vi "Start Continuous Output.vi"(0 "VISA resource name":refnum<visa-resource-name>, 7 "Continuous Measurement Type (Raw Accelerometer and Angular Rate)":u16(ring) items=["Raw Accelerometer and Angular Rate", "DeltaAngle & DeltaVelocity", "Orientation Matrix", "Orientation Update Matrix", "Acceleration, Angular Rate & Magnetometer Vectors", "Euler Angles", "Temperatures", "Gyro Stabilized Acceleration, Angular Rate & Magnetometer"], 11 "error in (no error)":errorcluster) -> (4 "VISA resource name out":refnum<visa-resource-name>, 15 "error out":errorcluster)   [LabVIEW 2012, in "MicroStrain 3DM-GXx.lvlib"]
doc: "Start continuous output of the specified measurement type."
uses:
  <instrlib>/MicroStrain 3DM-GXx/MicroStrain 3DM-GXx.lvlib
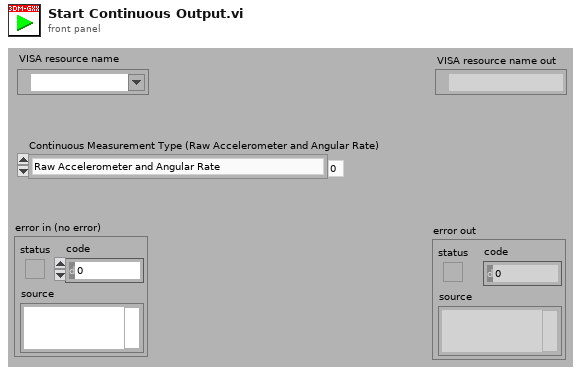
[diagram p1: front panel]
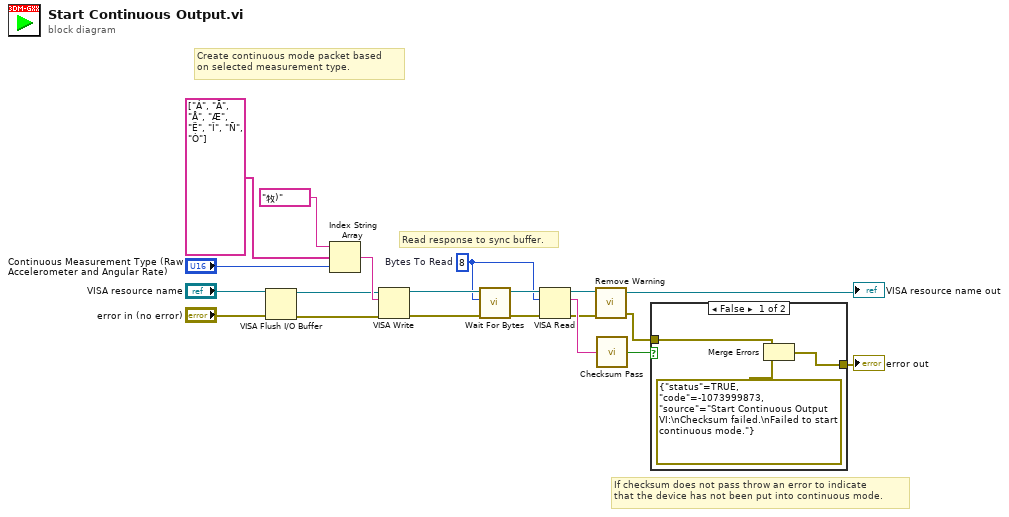
[diagram p0: block diagram]
diagram:
  w16 = u32 8  # Bytes To Read
  # "If checksum does not pass throw an error to indicate \nthat the device has not been put into continuous mode."
  # "Read response to sync buffer."
  # "Create continuous mode packet based \non selected measurement type."
  n1 = VISA Flush I/O Buffer(VISA resource name="VISA resource name", error in (no error)="error in (no error)") -> (VISA resource name out=w2:refnum<visa-resource-name>, error out=w1:errorcluster)  [unwired: 1 in]
  n2 = Index String Array(1:"Continuous Measurement Type (Raw Accelerometer and Angular Rate)", 2:string[] ["Á", "Ã", "Å", "Æ", "Ë", "Î", "Ñ", "Ò"] ("string array"), 3:"牧)" ("write buffer")) -> (0:w5:string)
  n3 = VISA Write(VISA resource name=w2, write buffer=w5, error in (no error)=w1) -> (VISA resource name out=w20:refnum<visa-resource-name>, error out=w19:errorcluster)  [unwired: 1 out]
  n4 = call <instrlib>:"Wait For Bytes.vi"("error in (no error)"=w19, "Bytes To Read (0)"=w16, "VISA resource name"=w20) -> ("error out"=w18:errorcluster, "VISA resource name out"=w17:refnum<visa-resource-name>)  [unwired: 7 in]
  n5 = VISA Read(VISA resource name=w17, byte count=w16, error in (no error)=w18) -> (VISA resource name out=w10:refnum<visa-resource-name>, read buffer=w15:string, error out=w11:errorcluster)  [unwired: 1 out]
  n6 = call <instrlib>:"Remove Warning.vi"("error in (no error)"=w11, "VISA resource name"=w10) -> ("error out"=w12:errorcluster, "VISA resource name out"=→"VISA resource name out":refnum<visa-resource-name>)  [unwired: 2 in]
  n7 = call <instrlib>:"Checksum Pass.vi"("Message In"=w15) -> ("Checksum Pass"=w14:bool)  [unwired: 4 in]
  n8 = case shown="False" w14 {
    tunnel: w12 -> [w23 w24]
    tunnel: [w22 w24] -> w13
    frame False {
      n9 = Merge Errors(w23, errorcluster {"status"=TRUE, "code"=-1073999873, "source"="Start Continuous Output VI:\nChecksum failed.\nFailed to start continuous mode."} ("error in 2 (no error)")) -> (w22:errorcluster)
    }
    frame True {
    }
  }
  "error out" <- w13
